vi "Set Content-Type.vi"(8 "error in (no error)":errorcluster, 10 "Content-Type":string, 11 "Gmail in":refnum<class "Gmail.lvclass">) -> (0 "error out":errorcluster, 3 "Gmail out":refnum<class "Gmail.lvclass">)   [LabVIEW 2020, in "Gmail API.lvlib" / "Gmail.lvclass"]
doc: "Sets the content-type for the email. In most circumstances this will be either \"text/plain\" or if sending HTML formatted content it should be \"text/html\" in order to be displayed correctly in email displays."
uses:
  Gmail.lvclass
  Gmail.lvclass/Gmail.ctl
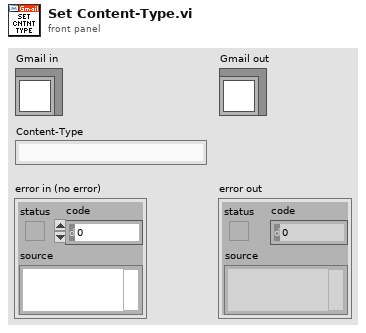
[diagram p1: front panel]
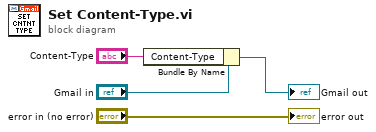
[diagram p0: block diagram]
diagram:
  n1 = Bundle By Name(cluster="Gmail in", "Content-Type"="Content-Type") -> (→"Gmail out":refnum<class "Gmail.lvclass">)
  "error out" <- "error in (no error)"
